vi "ScriptRequestVI.vi"(4 "Request Name":string, 5 "REPLYTypeDef Path":path, 6 "EventClusterName":string, 7 "REQTypeDef Path":path, 8 "error in (no error)":errorcluster, 10 "Module Ref":refnum<vi>, 11 "VI in":refnum<vi>) -> (0 "error out":errorcluster)   [LabVIEW 2024, in "AddNewEvent.lvlib"]
uses:
  Event/AddNewEvent.lvlib
  <vilib>/Utility/traverseref.llb/TRef TravTarget.ctl
panel:
  out "error out 2":errorcluster
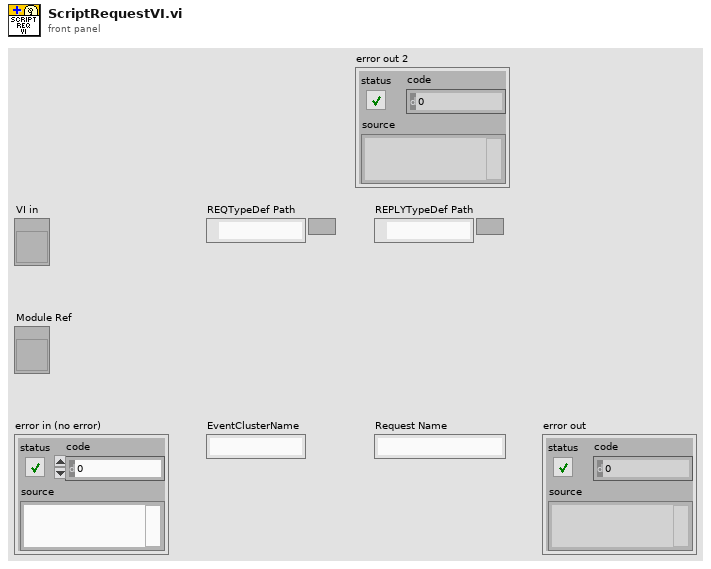
[diagram p1: front panel]
types:
  T1 = typedef "TRef TravTarget.ctl" = enum16{"FP", "BD", "Other"}
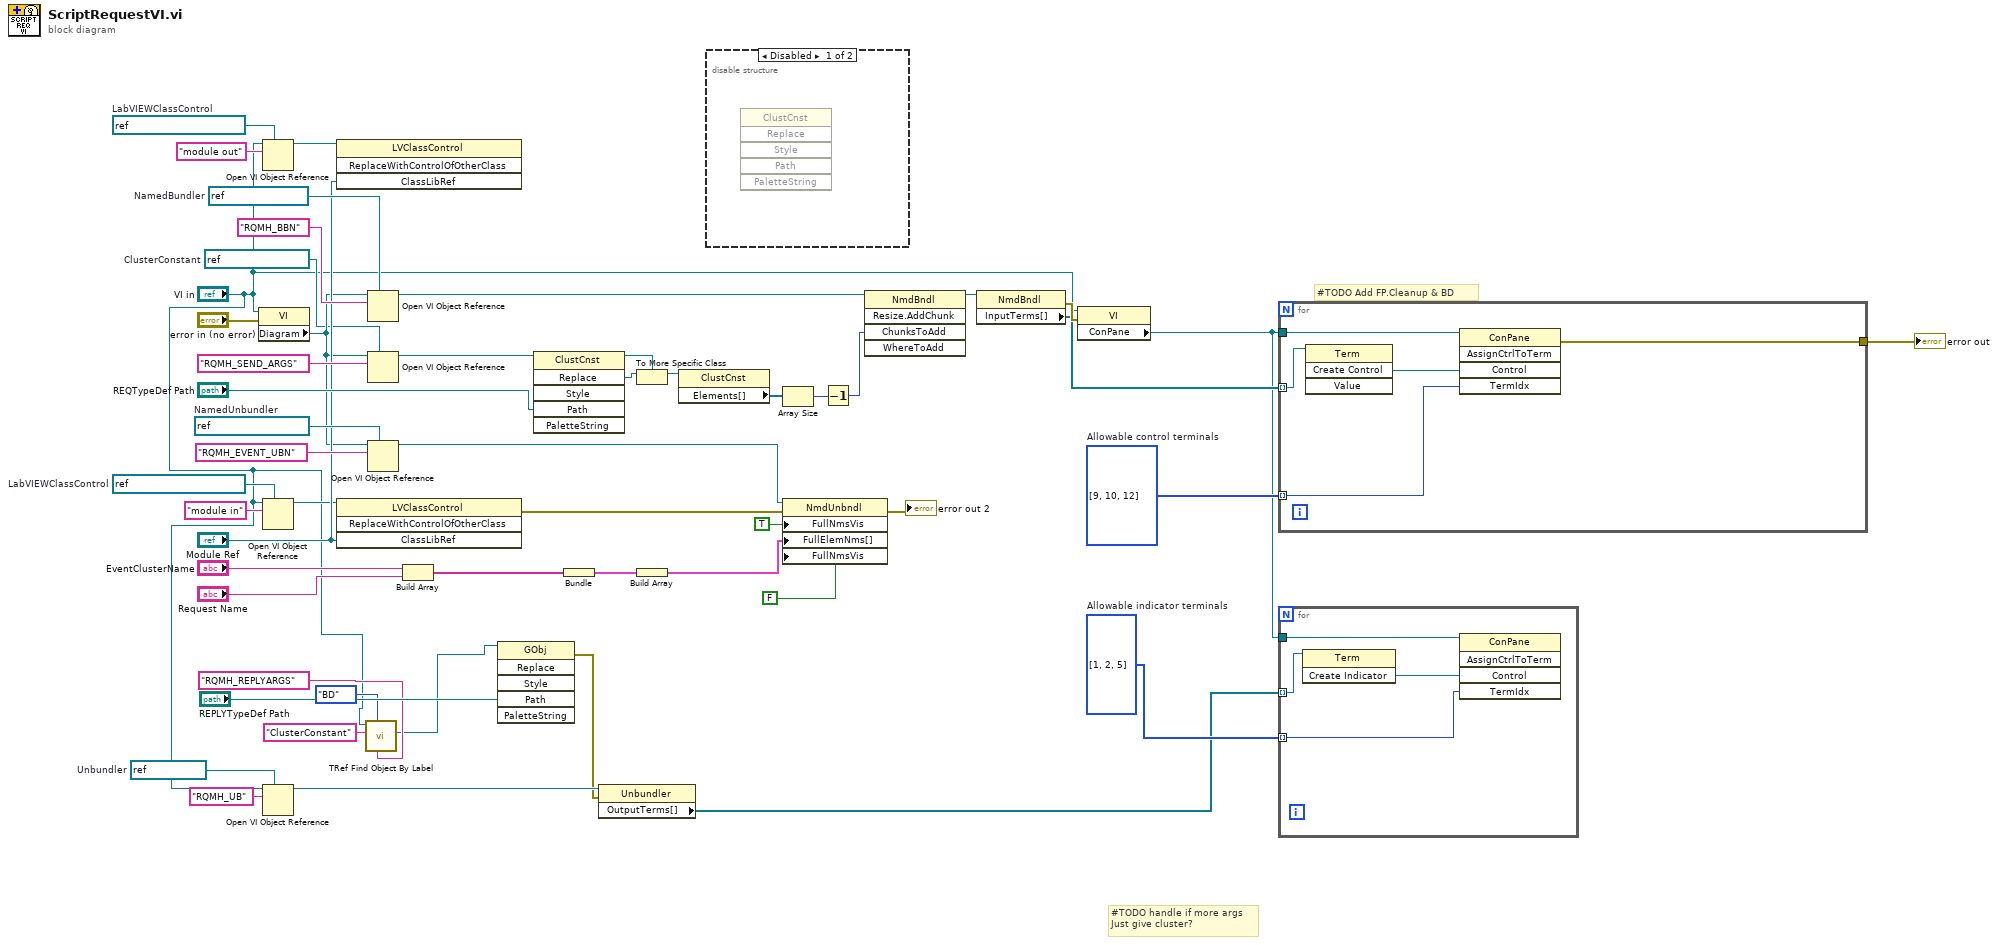
[diagram p0: block diagram]
diagram:
  w5 = i32[] [9, 10, 12]  # Allowable control terminals
  w4 = i32[] [1, 2, 5]  # Allowable indicator terminals
  w9 = refnum<vi> refnum  # Unbundler
  w31 = refnum<vi> refnum  # LabVIEWClassControl
  w28 = refnum<vi> refnum  # LabVIEWClassControl
  w11 = refnum<vi> refnum  # ClusterConstant
  w27 = refnum<vi> refnum  # NamedBundler
  w26 = refnum<vi> refnum  # NamedUnbundler
  # "#TODO handle if more args\nJust give cluster?"
  # "#TODO Add FP.Cleanup & BD"
  n1 = property class="VI"(reference="VI in", error in="error in (no error)") -> ("Diagram"=w17:refnum<vi>)  [unwired: 2 out]
  n2 = Open VI Object Reference(7:w31, 10:"module out" ("name/order"), 11:"VI in") -> (3:w32:refnum<vi>)  [unwired: 1 in, 1 out]
  n3 = Open VI Object Reference(7:w28, 10:"module in" ("name/order"), 11:"VI in") -> (3:w18:refnum<vi>)  [unwired: 1 in, 1 out]
  n4 = Open VI Object Reference(7:w9, 10:"RQMH_UB" ("name/order"), 11:"VI in") -> (3:w6:refnum<vi>)  [unwired: 1 in, 1 out]
  n5 = invoke class="LVClassControl" method="ReplaceWithControlOfOtherClass"(reference=w32, "ClassLibRef"="Module Ref") -> ()  [unwired: 2 in, 4 out]
  n6 = invoke class="LVClassControl" method="ReplaceWithControlOfOtherClass"(reference=w18, "ClassLibRef"="Module Ref") -> (error out=w48:errorcluster)  [unwired: 2 in, 3 out]
  n7 = call <vilib>:"TRef Find Object By Label.vi"("Label"="RQMH_REPLYARGS" ("name/order"), "Traverse Target"=TRef_TravTarget."BD", "Class Name"="ClusterConstant", "VI Ref"="VI in") -> ("Found Obj Ref"=w13:refnum<vi>)  [unwired: 4 in, 3 out]
  n8 = Open VI Object Reference(7:w27, 10:"RQMH_BBN" ("name/order"), 11:w17) -> (3:w39:refnum<vi>)  [unwired: 1 in, 1 out]
  n9 = Open VI Object Reference(7:w11, 10:"RQMH_SEND_ARGS" ("name/order"), 11:w17) -> (3:w38:refnum<vi>)  [unwired: 1 in, 1 out]
  n10 = Open VI Object Reference(7:w26, 10:"RQMH_EVENT_UBN" ("name/order"), 11:w17) -> (3:w35:refnum<vi>)  [unwired: 1 in, 1 out]
  n11 = Build Array("EventClusterName", "Request Name") -> (w33:string[])
  n12 = invoke class="GObj" method="Replace"(reference=w13, "Path"="REPLYTypeDef Path") -> (error out=w1:errorcluster)  [unwired: 4 in, 5 out]
  n13 = invoke class="ClustCnst" method="Replace"(reference=w38, "Path"="REQTypeDef Path") -> (reference out=w44:refnum<vi>, "Replace"=w42:refnum<vi>)  [unwired: 4 in, 4 out]
  n14 = Bundle(w33) -> (w34:cluster{string[]})  [unwired: 1 in]
  n15 = property class="Unbundler"(reference=w6, error in=w1) -> ("OutputTerms[]"=w3:refnum<vi>[])  [unwired: 2 out]
  n16 = To More Specific Class(target class=w44, reference=w42) -> (specific class reference=w43:refnum<vi>)  [unwired: 1 in, 1 out]
  n17 = Build Array(w34) -> (w36:cluster{string[]}[])
  n18 = property class="ClustCnst"(reference=w43) -> ("Elements[]"=w40:refnum<vi>[])  [unwired: 1 in, 2 out]
  n19 = disable-structure shown="Disabled" {
    frame Disabled {
      n20 = invoke class="ClustCnst" method="Replace"() -> ()  [unwired: 6 in, 6 out]
    }
    frame Enabled {
    }
  }
  n21 = Array Size(array=w40) -> (size(s)=w41:i32)
  n22 = property class="NmdUnbndl"(reference=w35, error in=w48, "FullNmsVis"=TRUE ("Full Names Visible?"), "FullElemNms[]"=w36, "FullNmsVis"=FALSE ("Full Names Visible?")) -> (error out=→"error out 2":errorcluster)  [unwired: 1 out]
  n23 = Decrement(x=w41) -> (x-1=w45:i32)
  n24 = invoke class="NmdBndl" method="Resize.AddChunk"(reference=w39, "ChunksToAdd"=w45) -> (reference out=w46:refnum<vi>)  [unwired: 3 in, 4 out]
  n25 = property class="NmdBndl"(reference=w46) -> (error out=w51:errorcluster, "InputTerms[]"=w20:refnum<vi>[])  [unwired: 1 in, 1 out]
  n26 = property class="VI"(reference="VI in", error in=w51) -> ("ConPane"=w2:refnum<vi>)  [unwired: 2 out]
  n27 = for {
    tunnel: w2 -> [w57]
    tunnel: [w56] -> w47
    tunnel: w20 -> [w55] mode=indexing
    tunnel: w5 -> [w54] mode=indexing
    n28 = invoke class="Term" method="Create Control"(reference=w55) -> ("Create Control"=w53:refnum<vi>)  [unwired: 3 in, 3 out]
    n29 = invoke class="ConPane" method="AssignCtrlToTerm"(reference=w57, "Control"=w53, "TermIdx"=w54) -> (error out=w56:errorcluster)  [unwired: 2 in, 4 out]
  }
  "error out" <- w47
  n30 = for {
    tunnel: w2 -> [w61]
    tunnel: w3 -> [w59] mode=indexing
    tunnel: w4 -> [w58] mode=indexing
    n31 = invoke class="Term" method="Create Indicator"(reference=w59) -> ("Create Indicator"=w60:refnum<vi>)  [unwired: 2 in, 2 out]
    n32 = invoke class="ConPane" method="AssignCtrlToTerm"(reference=w61, "Control"=w60, "TermIdx"=w58) -> ()  [unwired: 2 in, 5 out]
  }
